vi "TCP Control App.vi"() -> ()   [LabVIEW 2013]
panel:
  out "Status":string
  in  "Close FP":bool
  in  "Modal VIs":i32(listbox)
  in  "App Instance:":u16(ring) caption="Application Instance" items=["Default Application Instance", "Task Manager.lvproj:My Computer"]
  in  "Get Modal VIs":bool
  in  "Get Application Instances":bool
  # "This application helps close any open modal VIs that are not closeable otherwise.\n\nClick Refresh to get all modal VIs in memory, in all application instances.\n\nSelect the VI that you want to close and click Close FP"
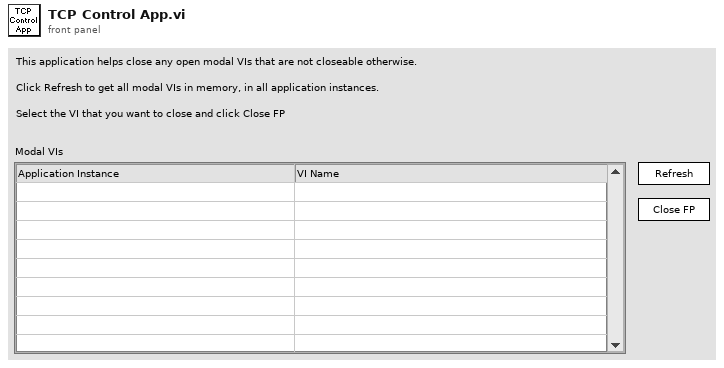
[diagram p1: front panel]
types:
  T1 = enum8{"Enabled", "Disabled", "Disabled and Grayed Out"}
  T2 = cluster{"connection ID":refnum<k5>, "buffer":string, "State":enum16{"Wait for connection", "Connected"}}
  T3 = enum16{"Standard", "Buffered", "CRLF", "Immediate"}
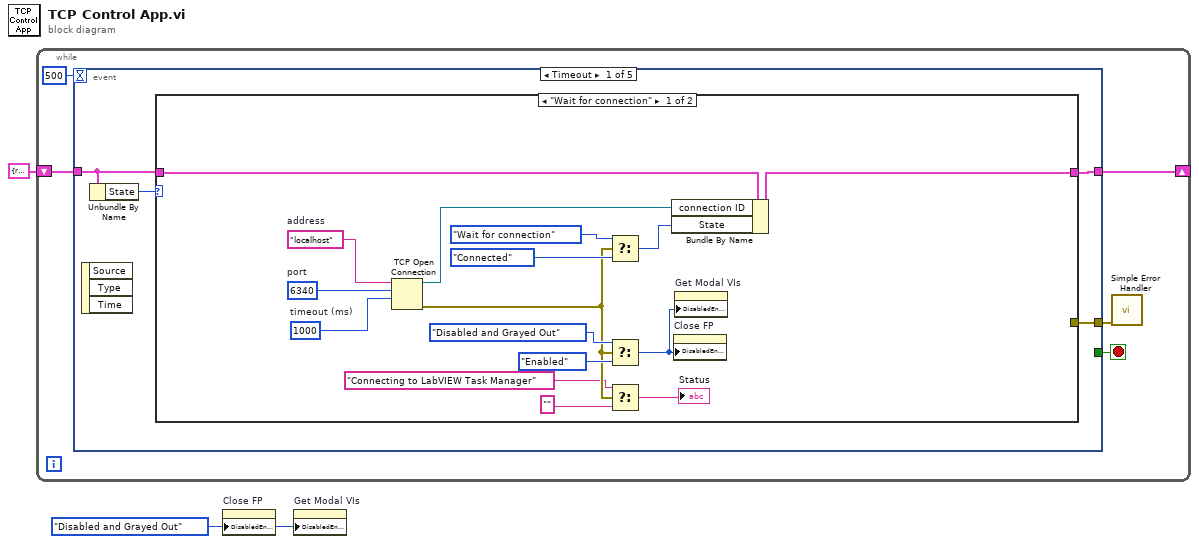
[diagram p0: block diagram]
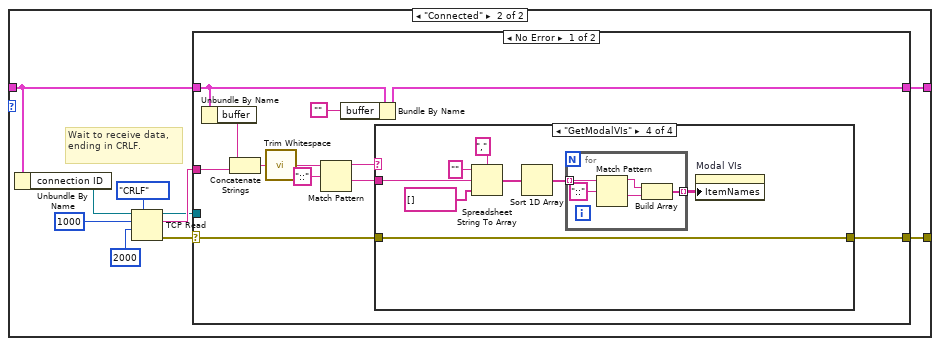
[diagram p2: hidden frame]
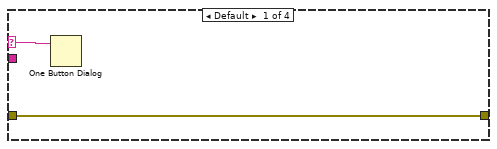
[diagram p3: hidden frame]
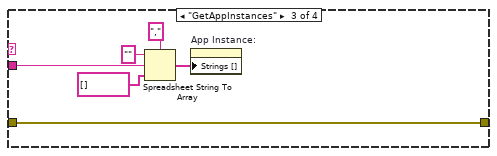
[diagram p5: hidden frame]
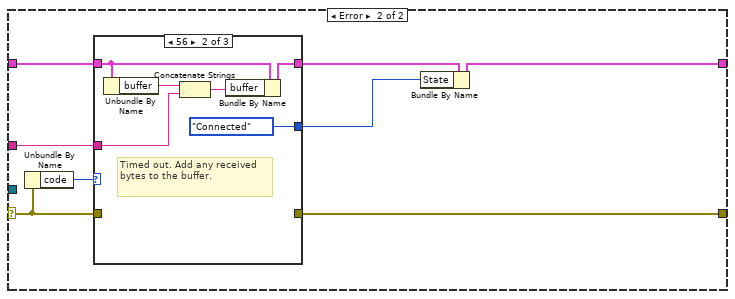
[diagram p6: hidden frame]
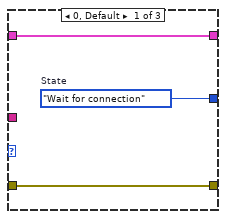
[diagram p7: hidden frame]
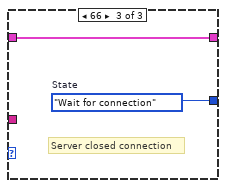
[diagram p8: hidden frame]
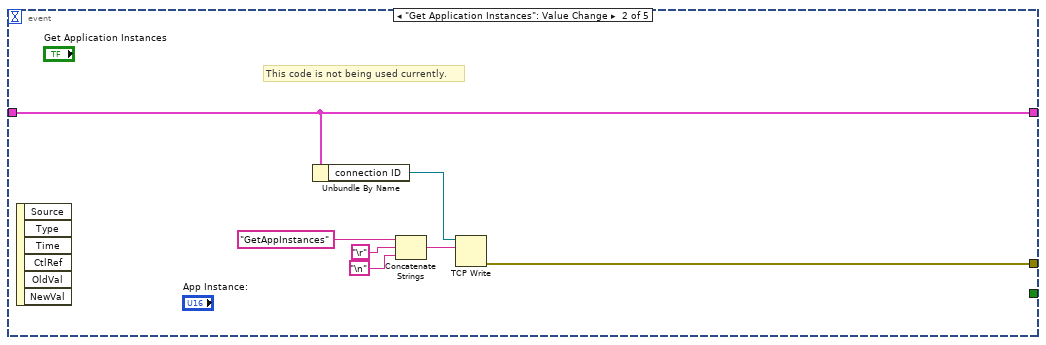
[diagram p9: hidden frame]
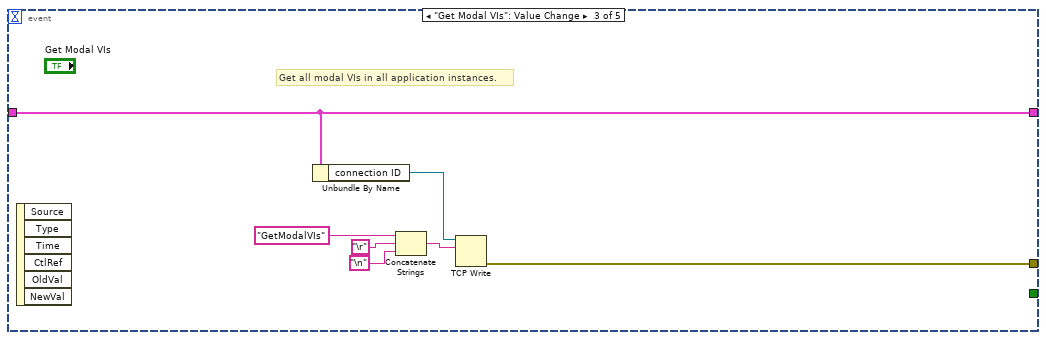
[diagram p10: hidden frame]
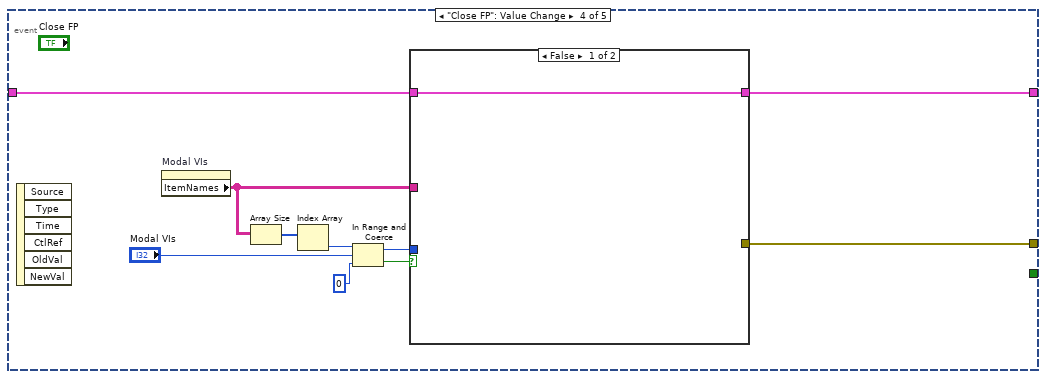
[diagram p11: hidden frame]
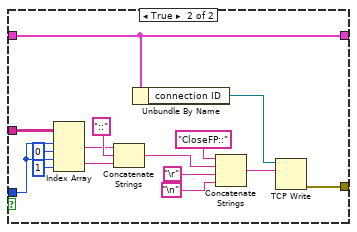
[diagram p12: hidden frame]
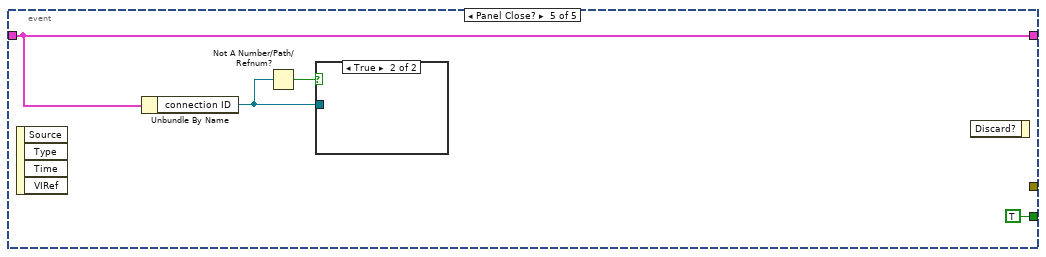
[diagram p13: hidden frame]
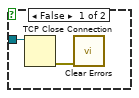
[diagram p14: hidden frame]
diagram:
  w1 = T1."Disabled and Grayed Out" ("Disabled")
  n1 = while {
    shift-right: [w7] -> _
    shift-left: T2 {"connection ID"=refnum, "buffer"="", "State"=enum."Wait for connection"} -> [w6]
    stop <- w5 stop-if-true
    n2 = event shown="[0] Timeout" {
      selector: _ -> [_ _ _ _ _]
      dyn-events: _ -> [_ _ _ _ _]
      timeout: 500 -> [_ _ _ _ _]
      tunnel: [w11 w93 w100 w105 w131] -> w7
      tunnel: w6 -> [w10 w93 w100 w114 w131]
      tunnel: [_ _ _ _ TRUE] -> w5
      tunnel: [w8 w91 w98 w113 _] -> w4
      event Timeout {
        n3 = event-data() -> ()  [unwired: 1 in, 3 out]
        n4 = Unbundle By Name(w10) -> ("State"=w9:enum16{"Wait for connection", "Connected"})
        n5 = case shown="\"Wait for connection\"" w9 {
          tunnel: [w27 w28] -> w11
          tunnel: w10 -> [w26 w29]
          tunnel: [_ w31] -> w8
          frame "Wait for connection" {
            w22 = 1000  # timeout (ms)
            w24 = u16 6340  # port
            w25 = "localhost"  # address
            n6 = TCP Open Connection(address=w25, remote port or service name=w24, timeout ms (60000)=w22) -> (connection ID=w23:refnum<k5>, error out=w15:errorcluster)  [unwired: 2 in]
            n7 = Select(t=enum16{"Wait for connection", "Connected"}."Wait for connection" ("State"), s=w15, f=enum16{"Wait for connection", "Connected"}."Connected" ("State")) -> (s? t:f=w19:enum16{"Wait for connection", "Connected"})
            n8 = Select(t=T1."Disabled and Grayed Out" ("Disabled"), s=w15, f=T1."Enabled" ("Disabled")) -> (s? t:f=w16:T1)
            n9 = Select(t="Connecting to LabVIEW Task Manager" ("Status"), s=w15, f="" ("Status")) -> (s? t:f=→"Status":string)
            n10 = Bundle By Name(cluster=w26, "connection ID"=w23, "State"=w19) -> (w27:T2)
            n11 = property on="Close FP" class="Bool"("DisabledEnum"=w16) -> ()  [unwired: 2 in, 2 out]
            n12 = property on="Get Modal VIs" class="Bool"("DisabledEnum"=w16) -> ()  [unwired: 2 in, 2 out]
          }
          frame "Connected" {
            # "Wait to receive data, ending in CRLF."
            n13 = Unbundle By Name(w29) -> ("connection ID"=w35:refnum<k5>)
            n14 = TCP Read(connection ID=w35, bytes to read=1000, 7:T3."CRLF" ("mode (standard)"), 9:2000 ("timeout ms (25000)")) -> (connection ID out=w30:refnum<k5>, data out=w33:string, error out=w34:errorcluster)  [unwired: 1 in]
            n15 = case shown="No Error" w34 {
              selector: w34 -> [w43 w77]
              tunnel: w33 -> [w49 w74]
              tunnel: [w42 w78] -> w31
              tunnel: w30 -> [_ _]
              tunnel: w29 -> [w47 w75]
              tunnel: [w45 w73] -> w28
              frame No Error {
                n16 = Unbundle By Name(w47) -> ("buffer"=w46:string)
                n17 = Concatenate Strings(w46, w49) -> (w48:string)
                n18 = call <vilib>:"Trim Whitespace.vi"("string"=w48) -> ("trimmed string"=w40:string)  [unwired: 1 in]
                n19 = Match Pattern(string=w40, regular expression="::") -> (before substring=w39:string, after substring=w38:string)  [unwired: 1 in, 2 out]
                n20 = Bundle By Name(cluster=w47, "buffer"="") -> (w45:T2)
                n21 = case shown="\"GetModalVIs\"" w39 {
                  selector: w39 -> [w51 _ _ _]
                  tunnel: w43 -> [w50 w52 w53 w62]
                  tunnel: [w50 w52 w53 w62] -> w42
                  tunnel: w38 -> [_ _ w58 w66]
                  frame Default {
                    n22 = One Button Dialog(message=w51) -> ()  [unwired: 1 in, 1 out]
                  }
                  frame "" {
                  }
                  frame "GetAppInstances" {
                    n23 = Spreadsheet String To Array(delimiter (Tab)=",", format string="", spreadsheet string=w58, array type (2D Dbl)=string[] [] ("Strings []")) -> (array=w54:string[])
                    n24 = property on="App Instance:" class="Ring (strict)"("Strings []"=w54) -> ()  [unwired: 2 in, 2 out]
                  }
                  frame "GetModalVIs" {
                    n25 = Spreadsheet String To Array(delimiter (Tab)=",", format string="", spreadsheet string=w66, array type (2D Dbl)=string[] [] ("Strings []")) -> (array=w61:string[])
                    n26 = Sort 1D Array(array=w61) -> (sorted array=w59:string[])
                    n27 = for {
                      tunnel: w59 -> [w70] mode=indexing
                      tunnel: [w67] -> w60 mode=indexing
                      n28 = Match Pattern(string=w70, regular expression="::") -> (before substring=w69:string, after substring=w68:string)  [unwired: 1 in, 2 out]
                      n29 = Build Array(w69, w68) -> (w67:string[])
                    }
                    n30 = property on="Modal VIs" class="MCListbox (strict)"("ItemNames"=w60) -> ()  [unwired: 2 in, 2 out]
                  }
                }
              }
              frame Error {
                n31 = Unbundle By Name(w77) -> ("code"=w79:i32)
                n32 = case shown="56" w79 {
                  tunnel: [w82 _ _] -> w78
                  tunnel: w77 -> [w82 _ _]
                  tunnel: [w81 w88 w90] -> w76
                  tunnel: w75 -> [w81 w87 w90]
                  tunnel: w74 -> [_ w84 _]
                  tunnel: [w80 enum16{"Wait for connection", "Connected"}."Connected" ("State") w89] -> w72
                  frame 0, Default {
                    w80 = enum16{"Wait for connection", "Connected"}."Wait for connection"  # State
                  }
                  frame 56 {
                    # "Timed out. Add any received bytes to the buffer."
                    n33 = Unbundle By Name(w87) -> ("buffer"=w86:string)
                    n34 = Concatenate Strings(w86, w84) -> (w85:string)
                    n35 = Bundle By Name(cluster=w87, "buffer"=w85) -> (w88:T2)
                  }
                  frame 66 {
                    w89 = enum16{"Wait for connection", "Connected"}."Wait for connection"  # State
                    # "Server closed connection"
                  }
                }
                n36 = Bundle By Name(cluster=w76, "State"=w72) -> (w73:T2)
              }
            }
          }
        }
      }
      event "Get Application Instances": Value Change {
        # "This code is not being used currently."
        n37 = event-data() -> ()  [unwired: 1 in, 6 out]
        n38 = Unbundle By Name(w93) -> ("connection ID"=w92:refnum<k5>)
        n39 = Concatenate Strings("GetAppInstances" ("string"), "\r", "\n") -> (w97:string)
        n40 = TCP Write(connection ID=w92, data in=w97) -> (error out=w91:errorcluster)  [unwired: 2 in, 2 out]
      }
      event "Get Modal VIs": Value Change {
        # "Get all modal VIs in all application instances."
        n41 = event-data() -> ()  [unwired: 1 in, 6 out]
        n42 = Unbundle By Name(w100) -> ("connection ID"=w99:refnum<k5>)
        n43 = Concatenate Strings("GetModalVIs" ("string"), "\r", "\n") -> (w104:string)
        n44 = TCP Write(connection ID=w99, data in=w104) -> (error out=w98:errorcluster)  [unwired: 2 in, 2 out]
      }
      event "Close FP": Value Change {
        n45 = event-data() -> ()  [unwired: 1 in, 6 out]
        n46 = property on="Modal VIs" class="MCListbox (strict)"() -> ("ItemNames"=w106:string[][])  [unwired: 2 in, 2 out]
        n47 = Array Size(array=w106) -> (size(s)=w112:i32[])
        n48 = Index Array(array=w112) -> (element=w111:i32)  [unwired: 1 in]
        n49 = In Range and Coerce(upper limit=w111, x="Modal VIs", lower limit=0) -> (coerced(x)=w107:i32, In Range?=w108:bool)
        n50 = case shown="False" w108 {
          tunnel: w114 -> [w115 w116]
          tunnel: [_ w125] -> w113
          tunnel: w107 -> [_ w123]
          tunnel: w106 -> [_ w124]
          tunnel: [w115 w116] -> w105
          frame False {
          }
          frame True {
            n51 = Index Array(array=w124, index (row) #1=w123, index (col) #1=0 ("disabled index (col)"), index (row) #2=w123, index (col) #2=1 ("disabled index (col)")) -> (element #1=w119:string, element #2=w118:string)
            n52 = Concatenate Strings(w119, "::" ("string"), w118) -> (w117:string)
            n53 = Unbundle By Name(w116) -> ("connection ID"=w126:refnum<k5>)
            n54 = Concatenate Strings("CloseFP::" ("string"), w117, "\r", "\n") -> (w130:string)
            n55 = TCP Write(connection ID=w126, data in=w130) -> (error out=w125:errorcluster)  [unwired: 2 in, 2 out]
          }
        }
      }
      event Panel Close? {
        n56 = event-data() -> ()  [unwired: 1 in, 4 out]
        n57 = Unbundle By Name(w131) -> ("connection ID"=w133:refnum<k5>)
        n58 = Not A Number/Path/Refnum?(number/path/refnum=w133) -> (NaN/Path/Refnum?=w132:bool)
        n59 = case shown="True" w132 {
          tunnel: w133 -> [w135 _]
          frame False {
            n60 = TCP Close Connection(connection ID=w135) -> (error out=w136:errorcluster)  [unwired: 1 in, 2 out]
            n61 = call <vilib>:"Clear Errors.vi"("error in (no error)"=w136) -> ()  [unwired: 6 in, 1 out]
          }
          frame True {
          }
        }
        n62 = event-data() -> ()  [unwired: 2 in, 1 out]
      }
    }
    n63 = call <vilib>:"Simple Error Handler.vi"("error in (no error)"=w4) -> ()  [unwired: 4 in, 5 out]
  }
  n64 = property on="Close FP" class="Bool"("DisabledEnum"=w1) -> ()  [unwired: 2 in, 2 out]
  n65 = property on="Get Modal VIs" class="Bool"("DisabledEnum"=w1) -> ()  [unwired: 2 in, 2 out]
